vi "Global Light Sensor.vi"() -> ()   [LabVIEW 2017]
panel:
  out "Red Light Sensed":bool
  out "Green Light Sensed":bool
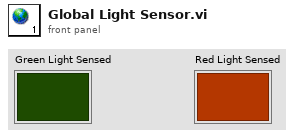
[diagram p1: front panel]
diagram:
